vi "lowLevelControllerQueueFGV.vi"(8 "error in (no error)":errorcluster, 11 "?":T1) -> (0 "error out":errorcluster, 3 "queue out":refnum<queue>)   [LabVIEW 2017, in "lowLevelController.lvlib"]
uses:
  lowLevelController.lvlib
  TypeDefs/queueFGVState.ctl
  TypeDefs/message.ctl
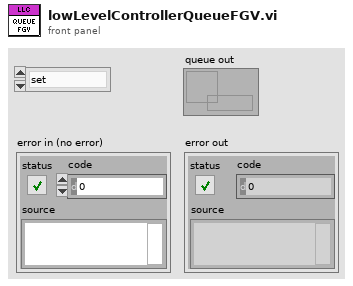
[diagram p1: front panel]
types:
  T1 = typedef "lowLevelController.lvlib/queueFGVState.ctl" = enum16{"set", "get"}
  T2 = typedef "lowLevelController.lvlib/message.ctl" = cluster{"calling module":string, "message":string, "data":variant}
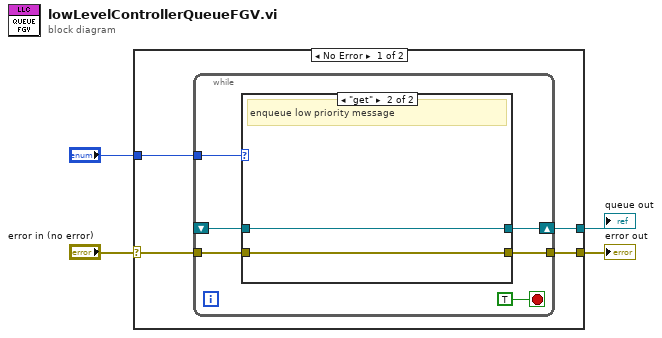
[diagram p0: block diagram]
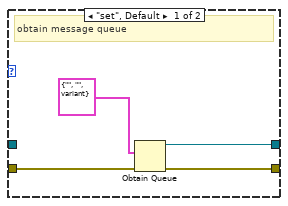
[diagram p2: hidden frame]
diagram:
  n1 = case shown="No Error" "error in (no error)" {
    selector: "error in (no error)" -> [w7 w21]
    tunnel: [w6 w21] -> w3
    tunnel: "?" -> [w8 _]
    tunnel: [w5 _] -> w1
    frame No Error {
      n2 = while {
        tunnel: w8 -> [w13]
        tunnel: w7 -> [w12]
        tunnel: [w11] -> w6
        shift-right: [w10] -> w5
        shift-left: _ -> [w9]
        stop <- TRUE stop-if-true
        n3 = case shown="\"get\"" w13 {
          tunnel: w12 -> [w18 w20]
          tunnel: [w17 w20] -> w11
          tunnel: [w16 w19] -> w10
          tunnel: w9 -> [_ w19]
          frame "set", Default {
            # "obtain message queue"
            n4 = Obtain Queue(element data type=T2 {"calling module"="", "message"="", "data"=variant}, error in (no error)=w18) -> (queue out=w16:refnum<queue>, error out=w17:errorcluster)  [unwired: 3 in, 1 out]
          }
          frame "get" {
            # "enqueue low priority message"
          }
        }
      }
    }
    frame Error {
    }
  }
  "error out" <- w3
  "queue out" <- w1
